vi "Sequence.CountersFglb.vi"(7 "Action (get)":T2=enum."get", 8 "error in":errorcluster, 9 "Init counters (0)":T1, 10 "Limit in failures":u16, 11 "Expected":u16) -> (0 "error out":errorcluster, 1 "Counters":T1, 2 "Partial order done":bool, 3 "Failures exceeded limit":bool)   [LabVIEW 2016]
uses:
  Sequence.CountersFglb.Action.ctl
  Sequence.Counters.ctl
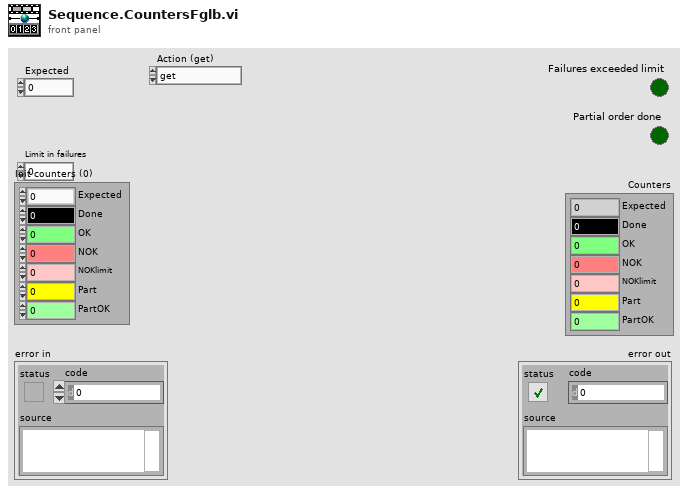
[diagram p1: front panel]
types:
  T1 = typedef "Sequence.Counters.ctl" = cluster{"Expected":u16, "Done":u16, "OK":u16, "NOK":u16, "NOKlimit":u16, "Part":u16, "PartOK":u16}
  T2 = typedef "Sequence.CountersFglb.Action.ctl" = enum16{"init", "clear", "confirm", "get", "pass", "fail"}
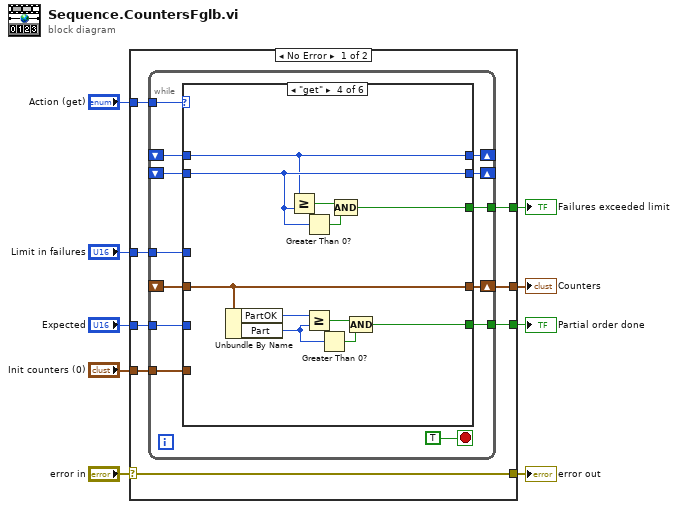
[diagram p0: block diagram]
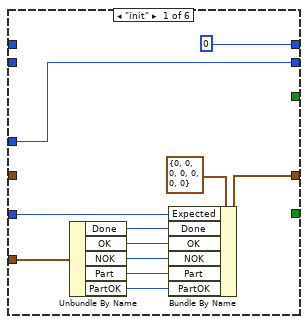
[diagram p2: hidden frame]
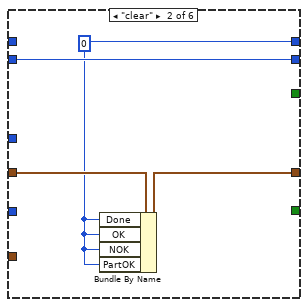
[diagram p3: hidden frame]
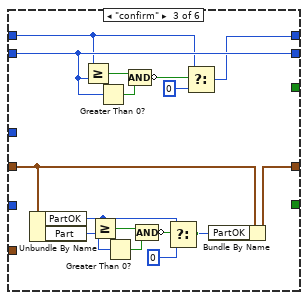
[diagram p4: hidden frame]
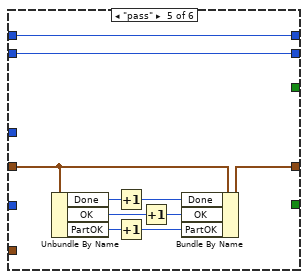
[diagram p5: hidden frame]
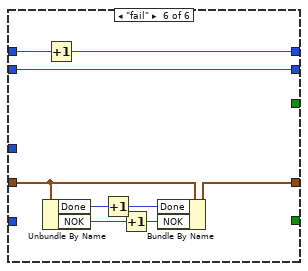
[diagram p6: hidden frame]
diagram:
  n1 = case shown="No Error" "error in" {
    selector: "error in" -> [w16 w92]
    tunnel: "Action (get)" -> [w17 _]
    tunnel: [w16 w92] -> w7
    tunnel: [w15 _] -> w6
    tunnel: "Expected" -> [w14 _]
    tunnel: "Limit in failures" -> [w13 _]
    tunnel: [w12 _] -> w3
    tunnel: "Init counters (0)" -> [w11 _]
    tunnel: [w10 _] -> w1
    frame No Error {
      n2 = while {
        tunnel: w17 -> [w29]
        shift-right: [w28] -> w15
        shift-left: _ -> [w27]
        tunnel: w14 -> [w26]
        shift-right: [w25] -> _
        shift-left: _ -> [w24]
        tunnel: w13 -> [w22]
        shift-right: [w23] -> _
        shift-left: _ -> [w21]
        tunnel: [w20] -> w12
        tunnel: w11 -> [w19]
        tunnel: [w18] -> w10
        stop <- TRUE stop-if-true
        n3 = case shown="\"get\"" w29 {
          tunnel: [w41 w44 w46 w67 w81 w90] -> w28
          tunnel: w27 -> [_ w45 w48 w67 w82 w91]
          tunnel: w26 -> [w40 _ _ _ _ _]
          tunnel: [u16 0 w42 w55 w68 w76 w84] -> w25
          tunnel: w24 -> [_ _ w57 w68 w76 w85]
          tunnel: [w39 w43 w59 w69 w77 w83] -> w23
          tunnel: w22 -> [w39 _ _ _ _ _]
          tunnel: w21 -> [_ w43 w59 w69 w77 w83]
          tunnel: [_ _ _ w70 _ _] -> w20
          tunnel: w19 -> [w37 _ _ _ _ _]
          tunnel: [_ _ _ w63 _ _] -> w18
          frame "init" {
            n4 = Unbundle By Name(w37) -> ("Done"=w36:u16, "OK"=w35:u16, "NOK"=w34:u16, "Part"=w32:u16, "PartOK"=w31:u16)
            n5 = Bundle By Name(cluster=T1 {"Expected"=0, "Done"=0, "OK"=0, "NOK"=0, "NOKlimit"=0, "Part"=0, "PartOK"=0} ("Counters"), "Expected"=w40, "Done"=w36, "OK"=w35, "NOK"=w34, "Part"=w32, "PartOK"=w31) -> (w41:T1)
          }
          frame "clear" {
            w42 = u16 0 ("Total")
            n6 = Bundle By Name(cluster=w45, "Done"=w42, "OK"=w42, "NOK"=w42, "PartOK"=w42) -> (w44:T1)
          }
          frame "confirm" {
            n7 = Unbundle By Name(w48) -> ("PartOK"=w47:u16, "Part"=w52:u16)
            n8 = Greater Or Equal?(x=w57, y=w59) -> (x >= y?=w61:bool)
            n9 = Greater Or Equal?(x=w47, y=w52) -> (x >= y?=w54:bool)
            n10 = Greater Than 0?(x=w59) -> (x > 0?=w60:bool)
            n11 = Greater Than 0?(x=w52) -> (x > 0?=w53:bool)
            n12 = Compound Arithmetic op=AND(w61, w60) -> (invert w58:bool)
            n13 = Compound Arithmetic op=AND(w54, w53) -> (invert w50:bool)
            n14 = Select(t=w47, s=w50, f=u16 0 ("Total")) -> (s? t:f=w49:u16)
            n15 = Select(t=w57, s=w58, f=u16 0 ("Total")) -> (s? t:f=w55:u16)
            n16 = Bundle By Name(cluster=w48, "PartOK"=w49) -> (w46:T1)
          }
          frame "get" {
            n17 = Unbundle By Name(w67) -> ("PartOK"=w62:u16, "Part"=w64:u16)
            n18 = Greater Or Equal?(x=w68, y=w69) -> (x >= y?=w72:bool)
            n19 = Greater Than 0?(x=w69) -> (x > 0?=w71:bool)
            n20 = Greater Or Equal?(x=w62, y=w64) -> (x >= y?=w66:bool)
            n21 = Greater Than 0?(x=w64) -> (x > 0?=w65:bool)
            n22 = Compound Arithmetic op=AND(w72, w71) -> (w70:bool)
            n23 = Compound Arithmetic op=AND(w66, w65) -> (w63:bool)
          }
          frame "pass" {
            n24 = Unbundle By Name(w82) -> ("Done"=w80:u16, "OK"=w79:u16, "PartOK"=w74:u16)
            n25 = Increment(x=w80) -> (x+1=w75:u16)
            n26 = Increment(x=w74) -> (x+1=w73:u16)
            n27 = Increment(x=w79) -> (x+1=w78:u16)
            n28 = Bundle By Name(cluster=w82, "Done"=w75, "OK"=w78, "PartOK"=w73) -> (w81:T1)
          }
          frame "fail" {
            n29 = Unbundle By Name(w91) -> ("Done"=w89:u16, "NOK"=w87:u16)
            n30 = Increment(x=w85) -> (x+1=w84:u16)
            n31 = Increment(x=w89) -> (x+1=w88:u16)
            n32 = Increment(x=w87) -> (x+1=w86:u16)
            n33 = Bundle By Name(cluster=w91, "Done"=w88, "NOK"=w86) -> (w90:T1)
          }
        }
      }
    }
    frame Error {
    }
  }
  "error out" <- w7
  "Counters" <- w6
  "Failures exceeded limit" <- w3
  "Partial order done" <- w1
